vi "Apply.vi"(8 "error in":errorcluster, 11 "DO DAQmx PWM Fixed Freq in":refnum<class "DO DAQmx Fixed Freq PWM CFG Simulated.lvclass">) -> (0 "error out":errorcluster, 3 "DO DAQmx PWM Fixed Freq out":refnum<class "DO DAQmx Fixed Freq PWM CFG Simulated.lvclass">)   [LabVIEW 2024, in "DAQmx Simulated CFGs.lvlib" / "DO DAQmx Fixed Freq PWM CFG Simulated.lvclass"]
uses:
  DO DAQmx Fixed Freq PWM CFG Simulated.lvclass
  Configurations/CFG Base/CFG Base.lvclass/CFG Base.ctl
  DO DAQmx Fixed Freq PWM CFG/DO DAQmx Fixed Freq PWM CFG.lvclass
  Configurations/CFG Base/CFG Base.lvclass
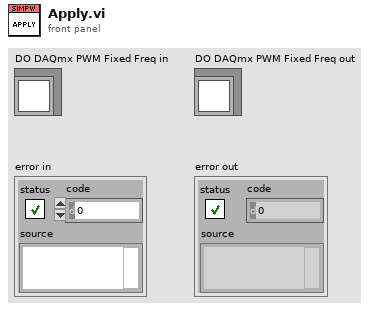
[diagram p1: front panel]
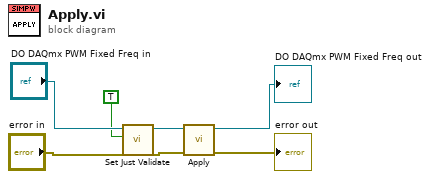
[diagram p0: block diagram]
diagram:
  n1 = call "Set Just Validate.vi"("Just Validate"=TRUE, "CFG Base in"="DO DAQmx PWM Fixed Freq in") -> ("CFG Base out"=w3:refnum<class "DO DAQmx Fixed Freq PWM CFG Simulated.lvclass">)  [unwired: 9 in]
  n2 = call-parent "Apply.vi"("error in"="error in", "DO DAQmx Fixed Freq PWM CFG in"=w3) -> ("error out"=→"error out":errorcluster, "DO DAQmx Fixed Freq PWM CFG out"=→"DO DAQmx PWM Fixed Freq out":refnum<class "DO DAQmx Fixed Freq PWM CFG Simulated.lvclass">)  [unwired: 8 in]
